vi "Refresh Memory.vi"(7 "Refresh?":bool, 8 "Error In":errorcluster, 11 "Refresh Programs Named":string) -> (0 "Error Out":errorcluster, 3 "Do not Robocopy":bool)   [LabVIEW 2016]
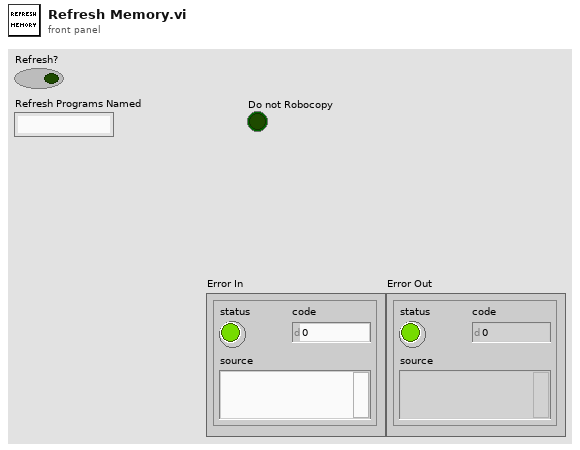
[diagram p1: front panel]
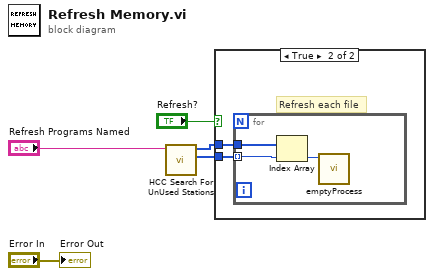
[diagram p0: block diagram]
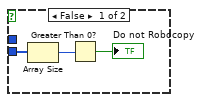
[diagram p2: hidden frame]
diagram:
  n1 = call "HCC Search For UnUsed Stations.vi"("Find Programs Named"="Refresh Programs Named") -> ("Array"=w4:i32[], "IDs 2"=w5:u32[])  [unwired: 6 in, 3 out]
  n2 = case shown="True" "Refresh?" {
    tunnel: w5 -> [_ w10]
    tunnel: w4 -> [w8 w9]
    frame False {
      n3 = Array Size(array=w8) -> (size(s)=w7:i32)
      n4 = Greater Than 0?(x=w7) -> (x > 0?=→"Do not Robocopy":bool)
    }
    frame True {
      # "Refresh each file"
      n5 = for {
        tunnel: w10 -> [w13]
        tunnel: w9 -> [w12] mode=indexing
        n6 = Index Array(array=w13, index=w12) -> (element=w11:u32)
        n7 = call "emptyProcess.vi"("ID"=w11) -> ()  [unwired: 11 out]
      }
    }
  }
  "Error Out" <- "Error In"
